vi "get_pos_no.vi"(4 "Status Old":dbl[][](array[numeric]), 5 "Array New Status":bool[](array[boolean]), 7 "Array Old Status":bool[](array[boolean])) -> (0 "Status New":dbl[][](array[numeric]), 2 "State":dbl, 3 "Position ID":dbl)   [LabVIEW 2021]
panel:
  out "Status Array Dim Init":dbl[][](array[numeric])
  out "Array":dbl[](array[numeric])
  out "State":bool
  out "Tray Row ID":dbl
  out "Tray Col ID":dbl
  out "New action":bool[](array[boolean])
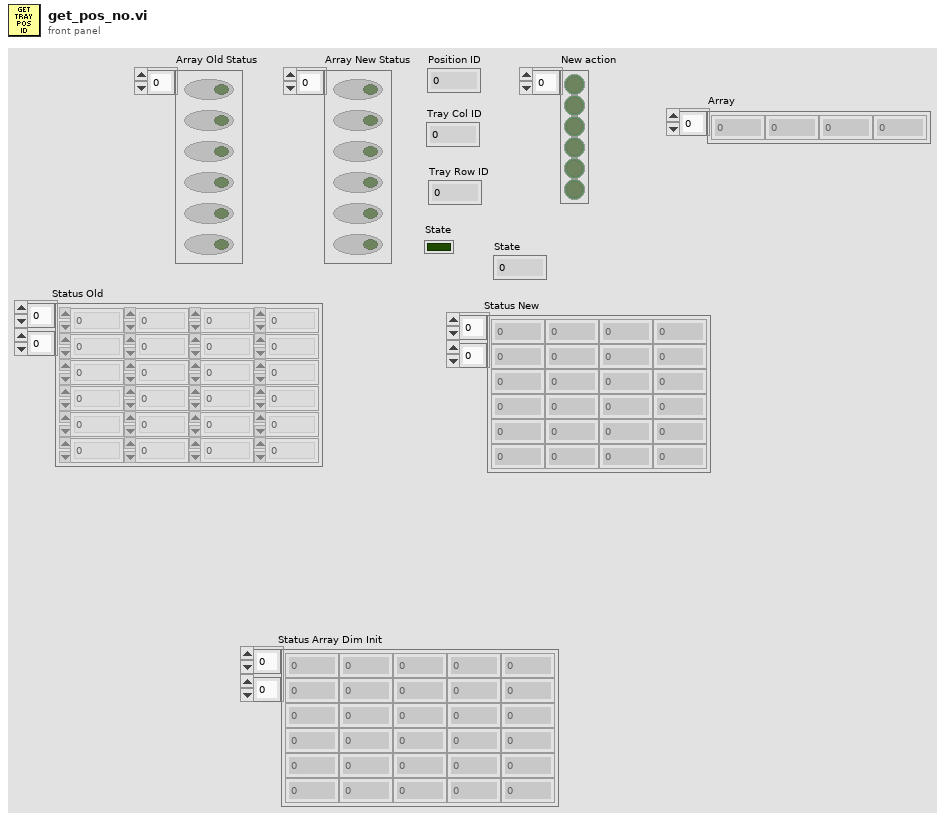
[diagram p1: front panel]
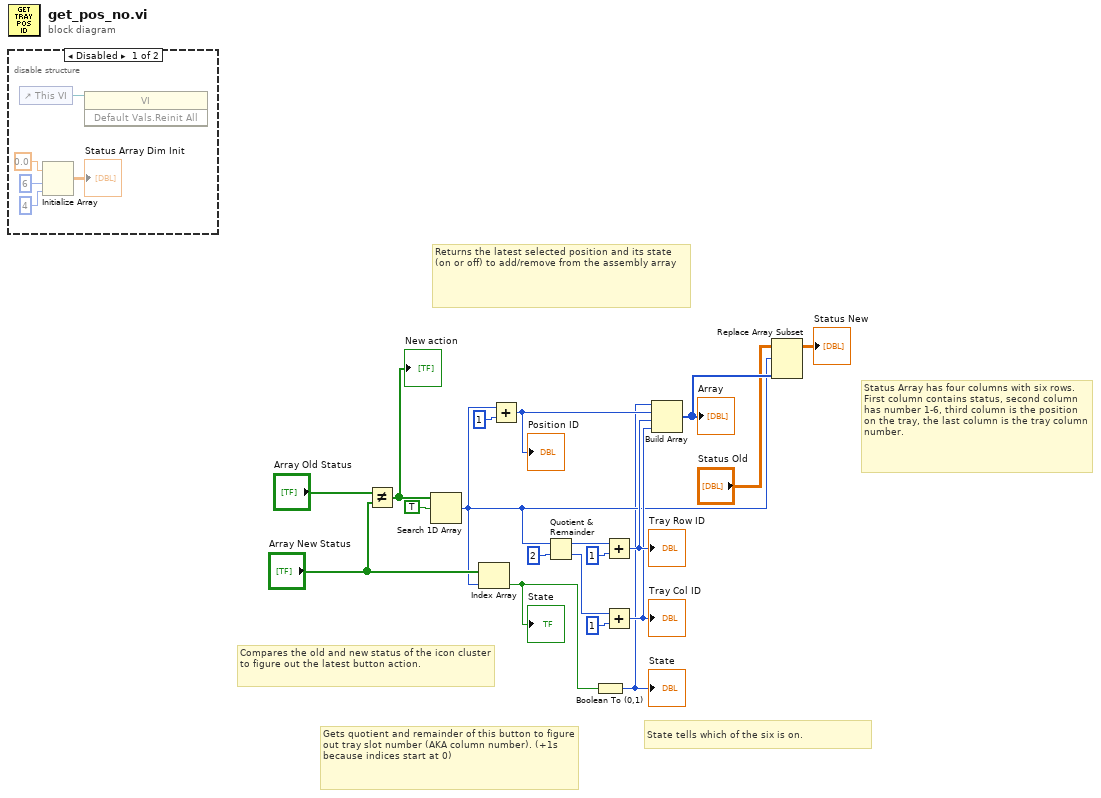
[diagram p0: block diagram]
diagram:
  # "Returns the latest selected position and its state (on or off) to add/remove from the assembly array"
  # "Status Array has four columns with six rows. First column contains status, second column has number 1-6, third column is the position on the tray, the last column is the tray column number."
  # "State tells which of the six is on."
  # "Gets quotient and remainder of this button to figure out tray slot number (AKA column number). (+1s because indices start at 0)"
  # "Compares the old and new status of the icon cluster to figure out the latest button action."
  n1 = disable-structure shown="Disabled" {
    frame Disabled {
      n2 = control-ref of="This VI"() -> (w24:refnum<vi>)
      n3 = Initialize Array(0.0 ("element"), 6 ("dimension size"), 4 ("dimension size")) -> (→"Status Array Dim Init":dbl[][])
      n4 = invoke class="VI" method="Default Vals.Reinit All"(reference=w24) -> ()  [unwired: 2 in, 3 out]
    }
    frame Enabled {
    }
  }
  n5 = Not Equal?(x="Array Old Status", y="Array New Status") -> (x != y?=w2:bool[])
  "New action" <- w2
  n6 = Search 1D Array(1D array=w2, element=TRUE) -> (index of element=w3:i32)  [unwired: 1 in]
  n7 = Index Array(array="Array New Status", index=w3) -> (element=w7:bool)
  "State" <- w7
  n8 = Add(x=w3, y=1) -> (x+y=w10:i32)
  "Position ID" <- w10
  n9 = Quotient & Remainder(x=w3, y=2) -> (x-y*floor(x/y)=w13:i32, floor(x/y)=w12:i32)
  n10 = Boolean To (0,1)(Boolean=w7) -> (0, 1=w1:i16)
  "State" <- w1
  n11 = Add(x=w13, y=1) -> (x+y=w9:i32)
  "Tray Row ID" <- w9
  n12 = Add(x=w12, y=1) -> (x+y=w8:i32)
  "Tray Col ID" <- w8
  n13 = Build Array(w1, w10, w9, w8) -> (w6:i32[])
  "Array" <- w6
  n14 = Replace Array Subset(array="Status Old", new element=w6, index (row)=w3) -> (→"Status New":dbl[][])  [unwired: 1 in]
